vi "WRP Setup Detector.vi"(8 "error in (no error)":errorcluster, 11 "detectorRegion":T1) -> (0 "error out":errorcluster, 2 "detectorRegionOut":T1, 3 "function return":i32)   [LabVIEW 2018, in "SesWrapper.lvlib"]
doc: "int STDCALL WRP_SetPropertyDouble(const String property, int index, const double *value);"
uses:
  SesWrapper.lvlib
  build/Debug/SESWrapper.dll
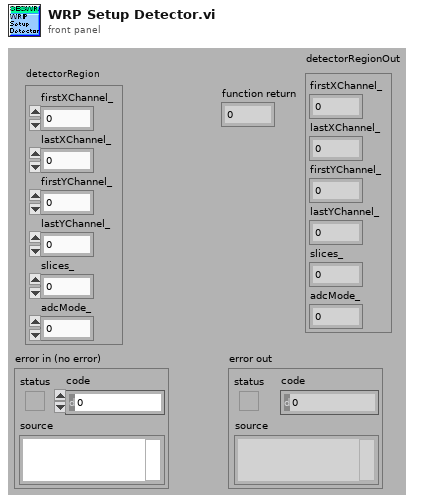
[diagram p1: front panel]
types:
  T1 = cluster{"firstXChannel_":i32, "lastXChannel_":i32, "firstYChannel_":i32, "lastYChannel_":i32, "slices_":i32, "adcMode_":u8}
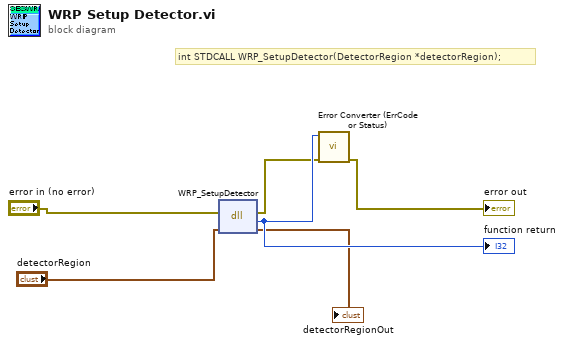
[diagram p0: block diagram]
diagram:
  # "int STDCALL WRP_SetupDetector(DetectorRegion *detectorRegion);"
  n1 = dll-call lib="C:/Development/svn/seswrapper-lib/build/Debug/SESWrapper.*" fn="WRP_SetupDetector" ("SESWrapper.dll:WRP_SetPropertyDouble")(error in="error in (no error)", "detectorRegion"="detectorRegion") -> (error out=w4:errorcluster, "return type"=w6:i32, "detectorRegion"=→"detectorRegionOut":T1)  [unwired: 2 in, 1 out]
  "function return" <- w6
  n2 = call "Error Converter (ErrCode or Status).vi"("error in (no error)"=w4, "error code"=w6) -> ("error out"=→"error out":errorcluster)  [unwired: 9 in]
